vi "Place piece.vi"(8 "error in (no error)":errorcluster, 9 "Piece":refnum<class "Piece.lvclass">, 10 "Destination":T1={"File"=enum."d", "Rank"=enum."4"}, 11 "Position in":refnum<class "Position.lvclass">) -> (0 "error out":errorcluster, 3 "Position out":refnum<class "Position.lvclass">)   [LabVIEW 2016, in "Chesslib.lvlib" / "Position.lvclass"]
uses:
  Position.lvclass
  typedef/Square.ctl
  typedef/File.ctl
  typedef/Rank.ctl
  Pieces/Piece/Piece.lvclass
  Position.lvclass/Position.ctl
  Board/Board.lvclass
  Chesslib.lvlib
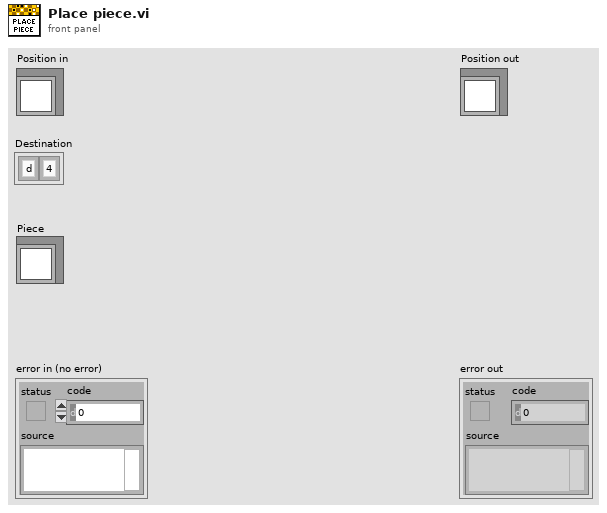
[diagram p1: front panel]
types:
  T1 = typedef "Chesslib.lvlib/Square.ctl" = cluster{"File":T2, "Rank":T3}
  T2 = typedef "Chesslib.lvlib/File.ctl" = enum8{"a", "b", "c", "d", "e", "f", "g", "h"}
  T3 = typedef "Chesslib.lvlib/Rank.ctl" = enum8{"1", "2", "3", "4", "5", "6", "7", "8"}
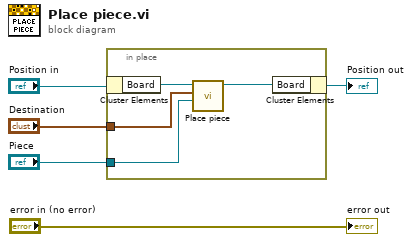
[diagram p0: block diagram]
diagram:
  n1 = in-place {
    in-place-border: "Destination" -> [w7]
    in-place-border: "Piece" -> [w6]
    n2 = in-place-cluster #1("Position in") -> ("Board"=w9:refnum<class "Board.lvclass">)
    n3 = call "Place piece.vi"("Piece"=w6, "Square"=w7, "Board in"=w9) -> ("Board out"=w8:refnum<class "Board.lvclass">)  [unwired: 6 in, 2 out]
    n4 = in-place-cluster #1("Board"=w8) -> (→"Position out":refnum<class "Position.lvclass">)
  }
  "error out" <- "error in (no error)"
